vi "Car Wash New.vi"() -> ()   [LabVIEW 2021]
uses:
  Controls/Car Wash Indicators.ctl
  Controls/Wash Options.ctl
  Controls/Time.ctl
panel:
  in  "stop":bool
  in  "Start":bool
  out "Elapsed Time":dbl format="%0.2f"
  out "Wash Entry":bool
  in  "Wash Options":T1
  in  "Car Position Slider":i32(slide) max=3 scale=0.0..4.0
  out "Car Wash Indicators":T2
  # "Entry Console"
  # "Car Wash Display"
  # "Car Position Simulation"
  # "Pre-Soak\nH-P Wash\nL-P Wax\nSpot Free Rinse"
  # "Underbody Wash\nBug Remover"
  # "Tire Shine\nAir Dry"
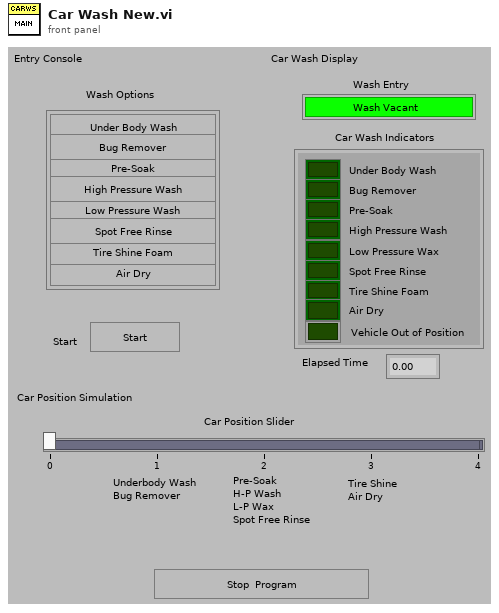
[diagram p1: front panel]
types:
  T1 = typedef "Wash Options.ctl" = cluster{"Underbody Wash":bool, "Bug Remover":bool, "Pre-Soak":bool, "High Pressure Wash":bool, "Low Pressure Wax":bool, "Spot Free Rinse":bool, "Tire Shine Foam":bool, "Air Dry":bool}
  T2 = typedef "Car Wash Indicators.ctl" = cluster{"Under Body Wash":bool, "Bug Remover":bool, "Pre-Soak":bool, "High Pressure Wash":bool, "Low Pressure Wax":bool, "Spot Free Rinse":bool, "Tire Shine Foam":bool, "Air Dry":bool, "Vehicle Out of Position":bool}
  T3 = enum32{"Invalid", "Standard", "Closed", "Hidden", "Minimized", "Maximized"}
  T4 = enum32{"invalid app kind", "Development System", "Run Time System", "Student Edition", "Embedded LabVIEW", "Evaluation", "Custom"}
  T5 = typedef "Time.ctl" = enum16{"Start", "Elapsed", "Pause", "int"}
  T6 = cluster{"Core":cluster{"Current VI Reference":refnum<vi>, "Close Panel on Exit?":bool}, "Your Boolean data":bool, "Your string data":string, "Wash Options":refnum<vi>, "Elapsed Time":refnum<vi>, "Car Position Slider":refnum<vi>, "Car Wash Indicators":refnum<vi>, "Wash Entry":refnum<vi>, "Time":dbl, "Car Wash Indicators":T2}
  T7 = cluster{"Current VI Reference":refnum<vi>, "Close Panel on Exit?":bool}
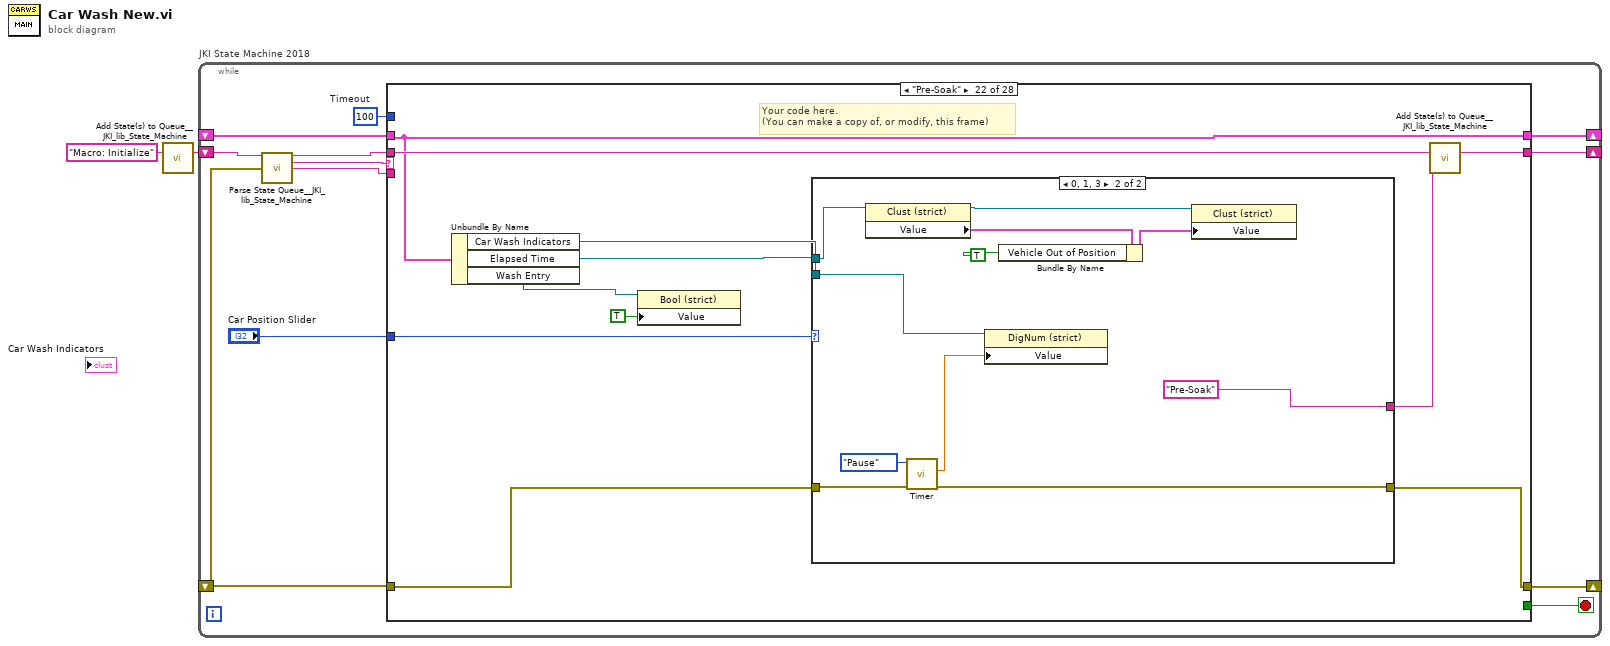
[diagram p0: block diagram]
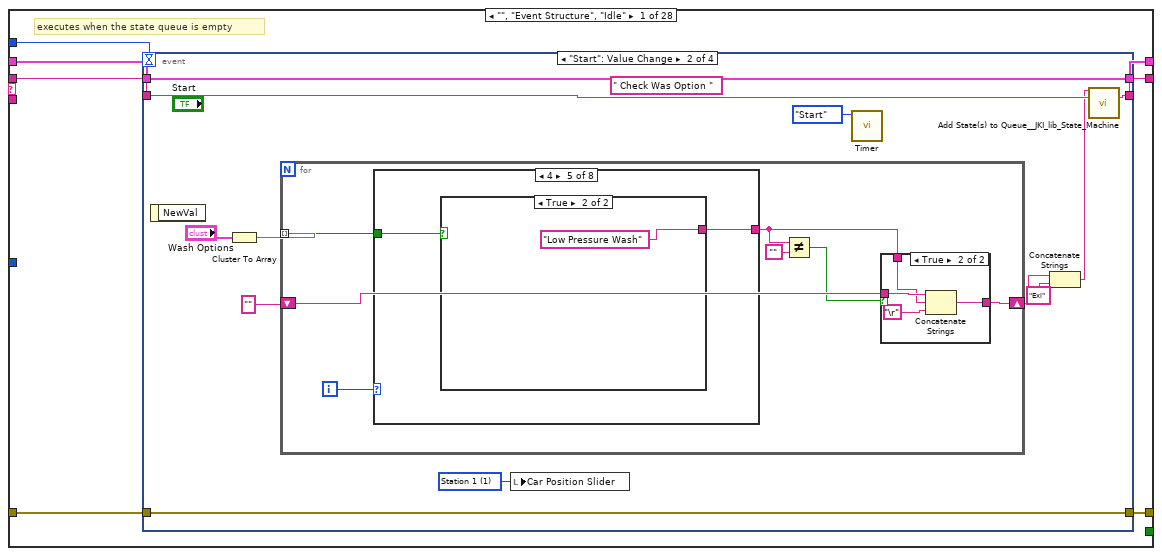
[diagram p2: hidden frame]
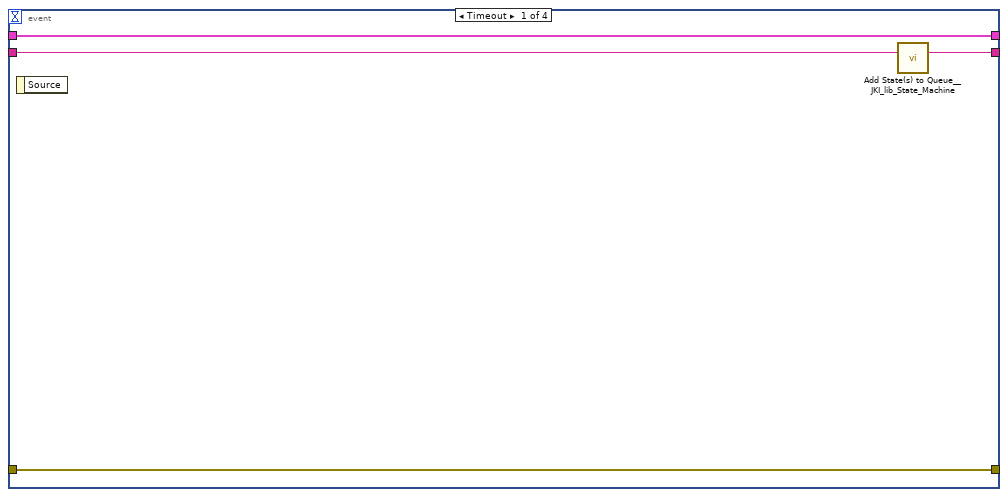
[diagram p3: hidden frame]
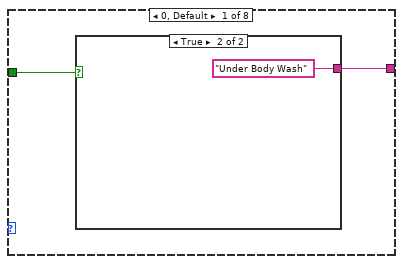
[diagram p5: hidden frame]
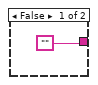
[diagram p6: hidden frame]
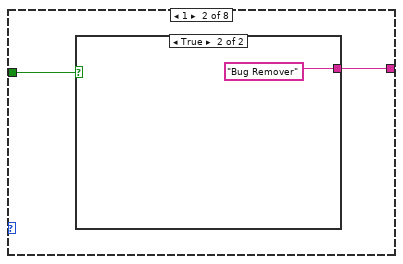
[diagram p7: hidden frame]
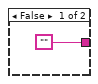
[diagram p8: hidden frame]
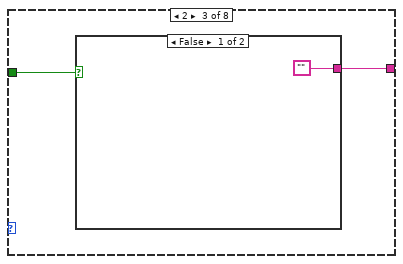
[diagram p9: hidden frame]
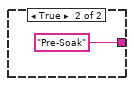
[diagram p10: hidden frame]
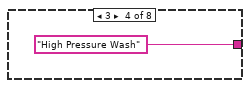
[diagram p11: hidden frame]
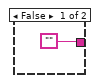
[diagram p12: hidden frame]
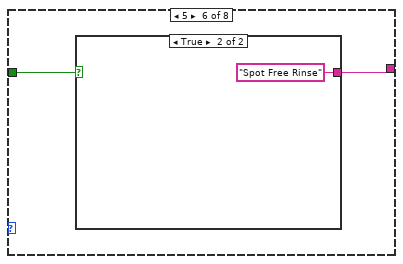
[diagram p13: hidden frame]
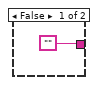
[diagram p14: hidden frame]
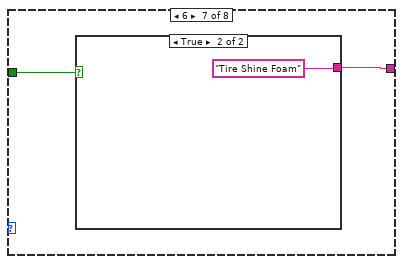
[diagram p15: hidden frame]
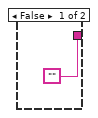
[diagram p16: hidden frame]
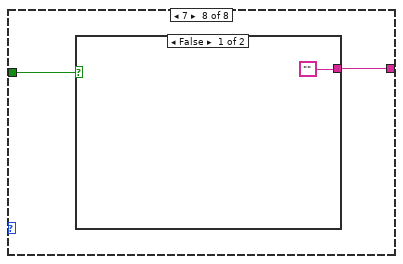
[diagram p17: hidden frame]
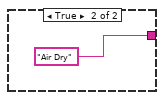
[diagram p18: hidden frame]
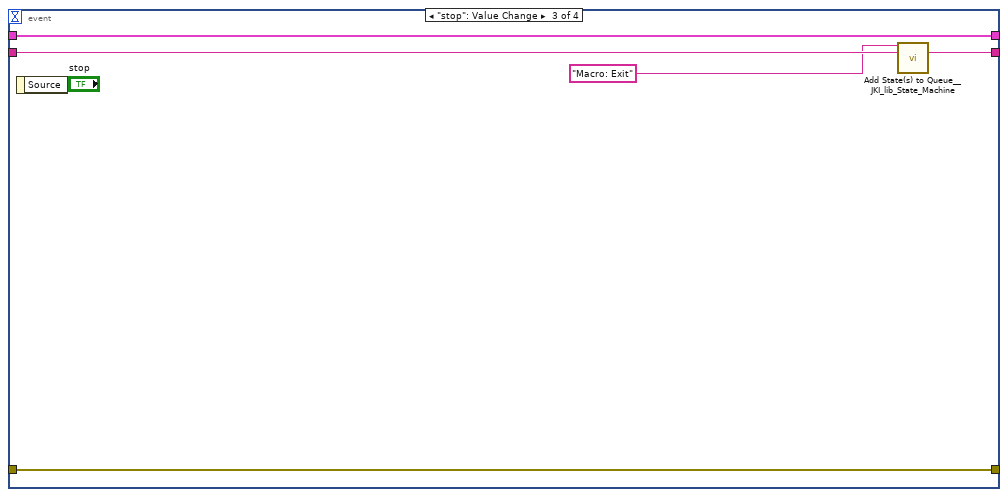
[diagram p19: hidden frame]
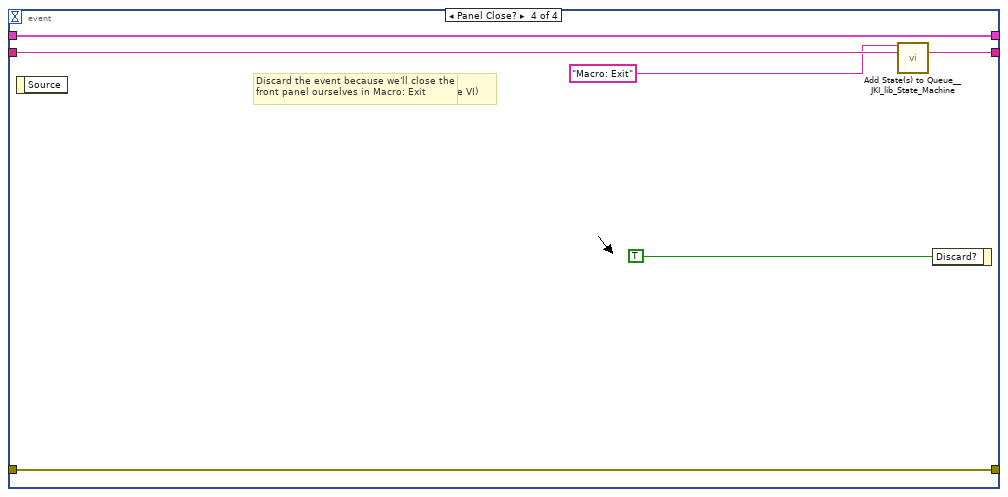
[diagram p20: hidden frame]
diagram:
  n1 = call <vilib>:"Add State(s) to Queue__JKI_lib_State_Machine.vi"("State(s) in (\"\")"="Macro: Initialize") -> ("States Out"=w2:string)  [unwired: 14 in]
  n2 = while "JKI State Machine 2018" {
    shift-right: [w7] -> _
    shift-left: _ -> [w3]
    shift-right: [w10] -> _
    shift-left: _ -> [w5]
    shift-right: [w9] -> _
    shift-left: w2 -> [w11]
    stop <- w8 stop-if-true
    w6 = 100  # Timeout
    n3 = call <vilib>:"Parse State Queue__JKI_lib_State_Machine.vi"("State Queue"=w11, "Error In (no error)"=w5) -> ("Remaining States"=w13:string, "Current State"=w14:string, "Arguments"=w12:string)  [unwired: 11 in]
    n4 = case shown="\"Pre-Soak\"" w14 {
      selector: w14 -> [_ _ w94 _ _ _ _ _ _ _ _ _ _ _ _ _ _ _ _ _ _ _ _ _ _ _ _ _]
      tunnel: w13 -> [w21 w93 w98 w117 w123 w128 w132 w148 w154 w158 w169 w175 w186 w255 w260 w270 w274 w278 w282 w293 w338 w383 w428 w473 w518 w563 w608 w652]
      tunnel: w12 -> [_ _ _ _ _ _ _ _ _ _ _ w170 w180 _ _ _ _ _ _ _ _ _ _ _ _ _ _ _]
      tunnel: w3 -> [w19 w90 w96 w110 w120 w126 w129 _ w149 w155 w160 w173 w182 w252 w257 w267 w271 w275 w279 w285 w330 w375 w420 w465 w510 w555 w600 w650]
      tunnel: [w18 w91 w100 w114 errorcluster {"status"=FALSE, "code"=0, "source"=""} ("error out") w125 w130 w145 w150 w156 w167 w171 w183 w253 w258 w268 w272 w276 w280 w288 w332 w380 w423 w469 w513 w558 w604 w647] -> w10
      tunnel: w5 -> [w17 w91 w99 w114 w119 w125 w130 w145 w151 w156 w167 w172 w184 w253 w258 w268 w272 w276 w280 w289 w333 w381 w425 w470 w514 w559 w605 w648]
      tunnel: [w20 w92 w97 w116 w122 w127 w131 w147 w153 w157 w168 w174 w185 w254 w259 w269 w273 w277 w281 w292 w337 w382 w427 w472 w517 w562 w607 w651] -> w9
      tunnel: [_ _ _ _ _ TRUE _ _ _ _ _ _ _ _ _ _ _ _ _ _ _ _ _ _ _ _ _ _] -> w8
      tunnel: [w16 w90 w96 w115 w120 w126 w129 w146 w149 w155 w160 w173 w182 w252 w257 w267 w271 w275 w279 w285 w330 w375 w420 w465 w510 w555 w600 w650] -> w7
      tunnel: w6 -> [w15 _ _ _ _ _ _ _ _ _ _ _ _ _ _ _ _ _ _ _ _ _ _ _ _ _ _ _]
      tunnel: "Car Position Slider" -> [_ _ _ _ _ _ _ _ _ _ _ _ _ _ _ _ _ _ _ w291 w334 w377 w422 w468 w515 w560 w603 w649]
      frame "", "Event Structure", "Idle" {
        # "executes when the state queue is empty"
        n5 = event shown="[1] \"Start\": Value Change" {
          selector: _ -> [_ _ _ _]
          dyn-events: _ -> [_ _ _ _]
          timeout: w15 -> [_ _ _ _]
          tunnel: w21 -> [w25 w37 w83 w89]
          tunnel: [w24 w36 w82 w88] -> w20
          tunnel: w19 -> [w22 w34 w80 w86]
          tunnel: [w23 w35 w81 w87] -> w18
          tunnel: w17 -> [w23 w35 w81 w87]
          tunnel: [w22 w34 w80 w86] -> w16
          event Timeout {
            n6 = event-data() -> ()  [unwired: 1 in, 1 out]
            n7 = call <vilib>:"Add State(s) to Queue__JKI_lib_State_Machine.vi"("State(s) in (\"\")"=w25) -> ("States Out"=w24:string)  [unwired: 14 in]
          }
          event "Start": Value Change {
            w26 = 1 items=["Entry", "Station 1", "Station 2", "Station 3", "Exit"] ("Car Position Slider")
            (unwired) " Check Was Option " ("State(s) at Back (\"\")")
            n8 = event-data() -> ()  [unwired: 1 in, 1 out]
            n9 = Cluster To Array(cluster="Wash Options") -> (array=w32:bool[])
            n10 = for {
              tunnel: w32 -> [w43] mode=indexing
              shift-right: [w42] -> w28
              shift-left: "" -> [w41]
              i -> [w44]
              n11 = case shown="4" w44 {
                tunnel: w43 -> [w51 w55 w59 _ w64 w68 w72 w76]
                tunnel: [w50 w54 w58 "High Pressure Wash" ("State(s) at Back (\"\")") w63 w67 w71 w75] -> w39
                frame 0, Default {
                  n12 = case shown="True" w51 {
                    tunnel: ["" "Under Body Wash" ("State(s) at Back (\"\")")] -> w50
                    frame False {
                    }
                    frame True {
                    }
                  }
                }
                frame 1 {
                  n13 = case shown="True" w55 {
                    tunnel: ["" "Bug Remover" ("State(s) at Back (\"\")")] -> w54
                    frame False {
                    }
                    frame True {
                    }
                  }
                }
                frame 2 {
                  n14 = case shown="False" w59 {
                    tunnel: ["" "Pre-Soak" ("State(s) at Back (\"\")")] -> w58
                    frame False {
                    }
                    frame True {
                    }
                  }
                }
                frame 3 {
                }
                frame 4 {
                  n15 = case shown="True" w64 {
                    tunnel: ["" "Low Pressure Wash" ("State(s) at Back (\"\")")] -> w63
                    frame False {
                    }
                    frame True {
                    }
                  }
                }
                frame 5 {
                  n16 = case shown="True" w68 {
                    tunnel: ["" "Spot Free Rinse"] -> w67
                    frame False {
                    }
                    frame True {
                    }
                  }
                }
                frame 6 {
                  n17 = case shown="True" w72 {
                    tunnel: ["" "Tire Shine Foam"] -> w71
                    frame False {
                    }
                    frame True {
                    }
                  }
                }
                frame 7 {
                  n18 = case shown="False" w76 {
                    tunnel: ["" "Air Dry"] -> w75
                    frame False {
                    }
                    frame True {
                    }
                  }
                }
              }
              n19 = Not Equal?(x=w39, y="") -> (x != y?=w38:bool)
              n20 = case shown="True" w38 {
                tunnel: [w45 w48] -> w42
                tunnel: w41 -> [w45 w47]
                tunnel: w39 -> [_ w46]
                frame False {
                }
                frame True {
                  n21 = Concatenate Strings(w47, w46, "\r") -> (w48:string)
                }
              }
            }
            n22 = local write "Car Position Slider"(w26) -> ()
            n23 = call "Timer.vi"("State"=enum16{"Start", "Elapsed", "Pause"}."Start") -> ()  [unwired: 8 in, 3 out]
            n24 = Concatenate Strings(w28, "Exi") -> (w27:string)
            n25 = call <vilib>:"Add State(s) to Queue__JKI_lib_State_Machine.vi"("State(s) in Front (\"\")"=w27, "State(s) in (\"\")"=w37) -> ("States Out"=w36:string)  [unwired: 13 in]
          }
          event "stop": Value Change {
            n26 = event-data() -> ()  [unwired: 1 in, 1 out]
            n27 = call <vilib>:"Add State(s) to Queue__JKI_lib_State_Machine.vi"("State(s) in Front (\"\")"="Macro: Exit", "State(s) in (\"\")"=w83) -> ("States Out"=w82:string)  [unwired: 13 in]
          }
          event Panel Close? {
            # "Discard the event because we'll close the front panel ourselves in Macro: Exit"
            # "Close Panel button (pressed) Event\n(this executes Macro: Exit to terminate the VI)"
            n28 = event-data() -> ()  [unwired: 1 in, 1 out]
            n29 = call <vilib>:"Add State(s) to Queue__JKI_lib_State_Machine.vi"("State(s) in Front (\"\")"="Macro: Exit", "State(s) in (\"\")"=w89) -> ("States Out"=w88:string)  [unwired: 13 in]
            n30 = event-data("Discard?"=TRUE) -> ()  [unwired: 1 in, 1 out]
          }
        }
      }
      frame "---------- Core ----------" {
        # "Do not put any code in this frame.\n(it is a separator no-op)"
        n31 = call <vilib>:"Add State(s) to Queue__JKI_lib_State_Machine.vi"("State(s) in (\"\")"=w93) -> ("States Out"=w92:string)  [unwired: 14 in]
      }
      frame Default {
        w103 = 42 items=["No error", "Argument error", "Memory is full", "Out of zone", "End of file", "File already open", "Generic file I/O error", "File not found", "File permission error", "Disk is full", "Duplicate path", "Too many files open", "System feature not enabled", "Resource file not found", "Cannot add resource", "Resource not found", "Image not found", "Image memory error", "Pen does not exist", "Config type invalid", "Config token not found", "Config parse error", "Config memory error", "Bad external code format", "Bad external code offset", "External code not present", "Null window", "Destroy window error", "Null menu", "Print aborted", "Bad print record", "Print driver error", "Windows error during printing", "Memory error during printing", "Print dialog error", "Generic print error", "Invalid device refnum", "Device not found", "Device parameter error", "Device unit error", "Cannot open device", "Device call aborted", "Generic error", "Cancelled by user", "Object ID too low", "Object ID too high", "Object not in heap", "Unknown heap", "Unknown object (invalid DefProc)", "Unknown object (DefProc not in table)", "Message out of range", "Invalid (null) method", "Unknown message", "Manager call not supported", "Bad address", "Network operation in progress", "Network operation timed out", "Connection is busy", "Network attribute not supported", "Network error", "Address in use", "System out of memory", "Connection aborted", "Connection refused", "Not connected", "Already connected", "Connection closed", "Initialization error (interapplication manager)", "Bad occurrence", "Wait on unbound occurrence handler", "Occurrence queue overflow", "Datalog type conflict", "Unused", "Unrecognized type (interapplication manager)", "Memory corrupt", "Failed to make temporary DLL", "Old CIN version", "Drag socket not found", "Failed to load drop-object", "Failed to register OLE object", "Failed to release OLE object", "Format specifier type mismatch", "Unknown format specifier", "Too few format specifiers", "Too many format specifiers", "Scan failed", "Newer CIN version", "Error converting to variant", "Runtime menu error", "Password tampered", "Variant attribute not found", "Incompatible variant data type", "Event data is not available", "Event Store is not present", "Occurrence is not found", "Event Queue is not created", "Event info is not available", "Refnum passed is NULL", "Error retrieving Class GUID", "Error retrieving CoClass GUID", "Error retrieving TypeLib GUID.", "Bad built application magic bytes.", "Specific driver is different from the specific driver associated with the Logical Name.", "There is no session opened to the class driver.", "Max Error", "MAX - Error with config objects", "MAX - Error loading configuration", "MAX - Group not supported"]
        # "Current State"
        # "Do not delete, rename, or modify this frame.\n(this is used to capture unhandled states and typos)"
        n32 = Format Into String(format string="Software Exception: Unhandled State \"%s\"." ("message"), error in=w99, w94) -> (resulting string=w102:string, error out=w101:errorcluster)  [unwired: 1 in]
        n33 = call <vilib>:"Error Cluster From Error Code.vi"("show call chain? (False)"=TRUE, "error in (no error)"=w101, "error message (\"\")"=w102, "error code (0)"=w103) -> ("error out"=w100:errorcluster)  [unwired: 5 in]
        n34 = call <vilib>:"Add State(s) to Queue__JKI_lib_State_Machine.vi"("State(s) in (\"\")"=w98) -> ("States Out"=w97:string)  [unwired: 14 in]
      }
      frame "Initialize Core Data" {
        # "Do not delete, rename, or modify this frame.\n(this is used to determine panel behavior on exit)"
        # "originally closed?"
        # "exe?"
        n35 = property class="VI"() -> ("FP.State"=w107:T3)  [unwired: 2 in, 2 out]
        n36 = property class="App"() -> ("App.Kind"=w113:T4)  [unwired: 2 in, 2 out]
        n37 = control-ref of="Current VI Reference"() -> (w108:refnum<vi>)
        n38 = Equal?(x=w107, y=T3."Closed" ("Front Panel Window:State")) -> (x = y?=w105:bool)
        n39 = Equal?(x=w113, y=T4."Run Time System" ("Application:Kind")) -> (x = y?=w111:bool)
        n40 = Or(x=w105, y=w111) -> (x .or. y?=w109:bool)
        n41 = Bundle By Name(cluster=w110, "Core.Current VI Reference"=w108, "Core.Close Panel on Exit?"=w109) -> (w115:T6)
        n42 = call <vilib>:"Add State(s) to Queue__JKI_lib_State_Machine.vi"("State(s) in (\"\")"=w117) -> ("States Out"=w116:string)  [unwired: 14 in]
      }
      frame "Error Handler" {
        # "Unhandled Error -- Display it"
        # "Handle any errors here.\nYou can also output any states to clean-up after errors occur"
        # "Clear error"
        n43 = call <vilib>:"General Error Handler.vi"("error in (no error)"=w119) -> ()  [unwired: 10 in, 5 out]
        n44 = call <vilib>:"Add State(s) to Queue__JKI_lib_State_Machine.vi"("State(s) in Front (\"\")"="/* Post Error States", "State(s) in (\"\")"=w123) -> ("States Out"=w122:string)  [unwired: 13 in]
      }
      frame "Exit" {
        # "Do not put any code in this frame.\n(No errors that occur here will be handled.)"
        n45 = call <vilib>:"Add State(s) to Queue__JKI_lib_State_Machine.vi"("State(s) in (\"\")"=w128) -> ("States Out"=w127:string)  [unwired: 14 in]
      }
      frame "---------- Data ----------" {
        # "Do not put any code in this frame.\n(It is a separator no-op. You can make a copy of this frame to create a new Data frame)"
        n46 = call <vilib>:"Add State(s) to Queue__JKI_lib_State_Machine.vi"("State(s) in (\"\")"=w132) -> ("States Out"=w131:string)  [unwired: 14 in]
      }
      frame "Data: Initialize" {
        w136 = 5.0  # Time
        w142 = T7 {"Current VI Reference"=refnum, "Close Panel on Exit?"=FALSE}  # Core
        w144 = TRUE  # Your Boolean data
        w143 = ""  # Your string data
        # "Initialize the shift-register data, here.\n(data names are defined by what you wire into the bundle function)"
        n47 = control-ref of="Elapsed Time"() -> (w141:refnum<vi>)
        n48 = control-ref of="Wash Options"() -> (w140:refnum<vi>)
        n49 = control-ref of="Car Position Slider"() -> (w139:refnum<vi>)
        n50 = control-ref of="Car Wash Indicators"() -> (w138:refnum<vi>)
        n51 = control-ref of="Wash Entry"() -> (w134:refnum<vi>)
        n52 = call "Timer.vi"("Timer (Sec)"=w136, "State"=Time."int") -> ()  [unwired: 7 in, 3 out]
        n53 = Bundle("Core"=w142, "Your Boolean data"=w144, "Your string data"=w143, "Wash Options"=w140, "Elapsed Time"=w141, "Car Position Slider"=w139, "Car Wash Indicators"=w138, "Wash Entry"=w134, "Time"=w136, "Car Wash Indicators"=T2 {"Under Body Wash"=FALSE, "Bug Remover"=FALSE, "Pre-Soak"=FALSE, "High Pressure Wash"=FALSE, "Low Pressure Wax"=FALSE, "Spot Free Rinse"=FALSE, "Tire Shine Foam"=FALSE, "Air Dry"=FALSE, "Vehicle Out of Position"=FALSE}) -> (w146:T6)  [unwired: 1 in]
        n54 = call <vilib>:"Add State(s) to Queue__JKI_lib_State_Machine.vi"("State(s) in (\"\")"=w148) -> ("States Out"=w147:string)  [unwired: 14 in]
        "Wash Entry" <- FALSE ("Wash Entry")
      }
      frame "Data: Cleanup" {
        # "Cleanup any data and references, here.\n(this is called automatically, by the Macro: Exit)"
        n55 = Unbundle By Name(w149) -> ("Core.Current VI Reference"=w152:refnum<vi>)
        n56 = Close Reference(reference=w152, error in (no error)=w151) -> (error out=w150:errorcluster)
        n57 = call <vilib>:"Add State(s) to Queue__JKI_lib_State_Machine.vi"("State(s) in (\"\")"=w154) -> ("States Out"=w153:string)  [unwired: 14 in]
      }
      frame "---------- UI ----------" {
        # "Do not put any code in this frame.\n(It is a separator no-op. You can make a copy of this frame to create a new UI frame)"
        n58 = call <vilib>:"Add State(s) to Queue__JKI_lib_State_Machine.vi"("State(s) in (\"\")"=w158) -> ("States Out"=w157:string)  [unwired: 14 in]
      }
      frame "UI: Initialize" {
        w159 = FALSE ("Car Wash Indicators.Under Body Wash")
        n59 = Unbundle By Name(w160) -> ("Car Wash Indicators"=w163:refnum<vi>, "Wash Entry"=w162:refnum<vi>)
        n60 = property class="Bool (strict)"(reference=w162, "Value"=FALSE) -> ()  [unwired: 1 in, 2 out]
        n61 = property class="Clust (strict)"(reference=w163) -> (reference out=w166:refnum<vi>, "Value"=w165:T2)  [unwired: 1 in, 1 out]
        n62 = Bundle By Name(cluster=w165, "Under Body Wash"=w159, "Bug Remover"=w159, "Pre-Soak"=w159, "High Pressure Wash"=w159, "Low Pressure Wax"=w159, "Spot Free Rinse"=w159, "Tire Shine Foam"=w159, "Air Dry"=w159, "Vehicle Out of Position"=w159) -> (w164:T2)
        n63 = property class="Clust (strict)"(reference=w166, "Value"=w164) -> ()  [unwired: 1 in, 2 out]
        n64 = call <vilib>:"Add State(s) to Queue__JKI_lib_State_Machine.vi"("State(s) in (\"\")"=w169) -> ("States Out"=w168:string)  [unwired: 14 in]
      }
      frame "UI: Cursor Set" {
        # "Argument"
        # "Set and Unset Cursor Busy.\n(Usage: \"UI: Cursor Set >> Busy|Idle\")"
        n65 = case shown="\"Idle\", Default" w170 {
          tunnel: w172 -> [w177 w179]
          tunnel: [w176 w178] -> w171
          frame "Idle", Default {
            n66 = call <vilib>:"Unset Busy.vi"("error in (no error)"=w177) -> ("error out"=w176:errorcluster)  [unwired: 10 in]
          }
          frame "Busy" {
            n67 = call <vilib>:"Set Busy.vi"("error in (no error)"=w179) -> ("error out"=w178:errorcluster)  [unwired: 9 in, 1 out]
          }
        }
        n68 = call <vilib>:"Add State(s) to Queue__JKI_lib_State_Machine.vi"("State(s) in (\"\")"=w175) -> ("States Out"=w174:string)  [unwired: 14 in]
      }
      frame "UI: Front Panel State" {
        # "Argument"
        # "Set Front Panel Open or Closed\n(Usage: \"UI: Front Panel State >> Open|Close\")"
        n69 = Unbundle By Name(w182) -> ("Core.Current VI Reference"=w181:refnum<vi>)
        n70 = case shown="\"Minimize\", \"Minimized\"" w180 {
          tunnel: w184 -> [w192 w207 w218 w231 w244]
          tunnel: [w194 w208 w220 w233 w246] -> w183
          tunnel: w181 -> [w193 w205 w219 w232 w245]
          frame "Open", "Standard", Default {
            w187 = T3."Standard" ("State")
            n71 = property class="VI"(reference=w193, error in=w192) -> (reference out=w190:refnum<vi>, error out=w191:errorcluster, "FP.State"=w189:T3)
            n72 = Not Equal?(x=w189, y=w187) -> (x != y?=w188:bool)
            n73 = case shown="True" w188 {
              tunnel: [w198 w200] -> w194
              tunnel: w191 -> [w197 w200]
              tunnel: w190 -> [w196 _]
              tunnel: w187 -> [w195 _]
              frame True {
                n74 = invoke class="VI" method="FP.Open"(reference=w196, error in=w197, "Activate"=TRUE, "State"=w195) -> (error out=w198:errorcluster)  [unwired: 1 in, 4 out]
              }
              frame False {
              }
            }
          }
          frame "Close", "Closed" {
            n75 = property class="VI"(reference=w205, error in=w207) -> (reference out=w204:refnum<vi>, error out=w206:errorcluster, "FP.State"=w202:T3)
            n76 = Not Equal?(x=w202, y=T3."Closed" ("Front Panel Window:State")) -> (x != y?=w201:bool)
            n77 = case shown="True" w201 {
              tunnel: [w209 w212] -> w208
              tunnel: w206 -> [w209 w211]
              tunnel: w204 -> [_ w210]
              frame False {
              }
              frame True {
                n78 = invoke class="VI" method="FP.Close"(reference=w210, error in=w211) -> (error out=w212:errorcluster)  [unwired: 1 in, 2 out]
              }
            }
          }
          frame "Hidden", "Hide" {
            w213 = T3."Hidden" ("State")
            n79 = property class="VI"(reference=w219, error in=w218) -> (reference out=w216:refnum<vi>, error out=w217:errorcluster, "FP.State"=w215:T3)
            n80 = Not Equal?(x=w215, y=w213) -> (x != y?=w214:bool)
            n81 = case shown="True" w214 {
              tunnel: [w224 w225] -> w220
              tunnel: w217 -> [w223 w225]
              tunnel: w216 -> [w222 _]
              tunnel: w213 -> [w221 _]
              frame True {
                n82 = invoke class="VI" method="FP.Open"(reference=w222, error in=w223, "State"=w221) -> (error out=w224:errorcluster)  [unwired: 2 in, 4 out]
              }
              frame False {
              }
            }
          }
          frame "Minimize", "Minimized" {
            w226 = T3."Minimized" ("State")
            n83 = property class="VI"(reference=w232, error in=w231) -> (reference out=w229:refnum<vi>, error out=w230:errorcluster, "FP.State"=w228:T3)
            n84 = Not Equal?(x=w228, y=w226) -> (x != y?=w227:bool)
            n85 = case shown="True" w227 {
              tunnel: [w237 w238] -> w233
              tunnel: w230 -> [w236 w238]
              tunnel: w229 -> [w235 _]
              tunnel: w226 -> [w234 _]
              frame True {
                n86 = invoke class="VI" method="FP.Open"(reference=w235, error in=w236, "State"=w234) -> (error out=w237:errorcluster)  [unwired: 2 in, 4 out]
              }
              frame False {
              }
            }
          }
          frame "Maximize", "Maximized" {
            w239 = T3."Maximized" ("State")
            n87 = property class="VI"(reference=w245, error in=w244) -> (reference out=w242:refnum<vi>, error out=w243:errorcluster, "FP.State"=w241:T3)
            n88 = Not Equal?(x=w241, y=w239) -> (x != y?=w240:bool)
            n89 = case shown="True" w240 {
              tunnel: [w250 w251] -> w246
              tunnel: w243 -> [w249 w251]
              tunnel: w242 -> [w248 _]
              tunnel: w239 -> [w247 _]
              frame True {
                n90 = invoke class="VI" method="FP.Open"(reference=w248, error in=w249, "State"=w247) -> (error out=w250:errorcluster)  [unwired: 2 in, 4 out]
              }
              frame False {
              }
            }
          }
        }
        n91 = call <vilib>:"Add State(s) to Queue__JKI_lib_State_Machine.vi"("State(s) in (\"\")"=w186) -> ("States Out"=w185:string)  [unwired: 14 in]
      }
      frame "---------- Macro ----------" {
        # "Do not put any code in this frame.\n(It is a separator no-op. You can make a copy of this frame to create a new Macro frame)"
        n92 = call <vilib>:"Add State(s) to Queue__JKI_lib_State_Machine.vi"("State(s) in (\"\")"=w255) -> ("States Out"=w254:string)  [unwired: 14 in]
      }
      frame "Macro: Initialize" {
        w256 = "Data: Initialize\nInitialize Core Data\nUI: Initialize\nUI: Front Panel State >> Open"  # Data: Initialize Initialize Core Data UI: Initialize UI: Front Panel State >> Open
        # "Initialization Macro\n(This is called once, when the VI starts)"
        n93 = call <vilib>:"Add State(s) to Queue__JKI_lib_State_Machine.vi"("State(s) in Front (\"\")"=w256, "State(s) in (\"\")"=w260) -> ("States Out"=w259:string)  [unwired: 13 in]
      }
      frame "Macro: Exit" {
        # "Exit Macro\n(This is called once, when the VI exits)"
        n94 = Unbundle By Name(w267) -> ("Core.Close Panel on Exit?"=w266:bool)
        n95 = Select(t="UI: Front Panel State >> Close", s=w266, f="") -> (s? t:f=w263:string)
        n96 = call <vilib>:"Add State(s) to Queue__JKI_lib_State_Machine.vi"("State(s) in (\"\")"=w263, "State(s) at Back (\"\")"="Data: Cleanup\nExit") -> ("States Out"=w261:string)  [unwired: 13 in]
        n97 = call <vilib>:"Add State(s) to Queue__JKI_lib_State_Machine.vi"("State(s) in Front (\"\")"=w261, "State(s) in (\"\")"=w270) -> ("States Out"=w269:string)  [unwired: 13 in]
      }
      frame "---------- New Category ----------" {
        # "Template Separator\n(You can make a copy of, or modify, this frame)"
        n98 = call <vilib>:"Add State(s) to Queue__JKI_lib_State_Machine.vi"("State(s) in (\"\")"=w274) -> ("States Out"=w273:string)  [unwired: 14 in]
      }
      frame "New Category: 1" {
        # "Your code here.\n(You can make a copy of, or modify, this frame)"
        n99 = call <vilib>:"Add State(s) to Queue__JKI_lib_State_Machine.vi"("State(s) in (\"\")"=w278) -> ("States Out"=w277:string)  [unwired: 14 in]
      }
      frame "New Category: 2" {
        # "Your code here.\n(You can make a copy of, or modify, this frame)"
        n100 = call <vilib>:"Add State(s) to Queue__JKI_lib_State_Machine.vi"("State(s) in (\"\")"=w282) -> ("States Out"=w281:string)  [unwired: 14 in]
      }
      frame "Under Body Wash" {
        # "Your code here.\n(You can make a copy of, or modify, this frame)"
        n101 = Unbundle By Name(w285) -> ("Car Wash Indicators"=w286:refnum<vi>, "Elapsed Time"=w290:refnum<vi>, "Wash Entry"=w283:refnum<vi>)
        n102 = property class="Bool (strict)"(reference=w283, "Value"=TRUE) -> ()  [unwired: 1 in, 2 out]
        n103 = case shown="1, Default" w291 {
          tunnel: [w306 w322] -> w288
          tunnel: w290 -> [w301 w326]
          tunnel: [w303 "Under Body Wash"] -> w287
          tunnel: w289 -> [w302 w323]
          tunnel: w286 -> [w297 w320]
          frame 1, Default {
            n104 = property class="Clust (strict)"(reference=w297) -> (reference out=w294:refnum<vi>, "Value"=w296:T2)  [unwired: 1 in, 1 out]
            n105 = call "Timer.vi"("entrée d'erreur"=w302, "State"=Time."Elapsed") -> ("sortie d'erreur"=w307:errorcluster, "Elapsed"=w300:dbl, "Elapsed?"=w308:bool)  [unwired: 7 in]
            n106 = property class="DigNum (strict)"(reference=w301, "Value"=w300) -> (reference out=w299:refnum<vi>)  [unwired: 1 in, 1 out]
            n107 = Bundle By Name(cluster=w296, "Vehicle Out of Position"=FALSE, "Under Body Wash"=TRUE) -> (w295:T2)
            n108 = case shown="False" w308 {
              tunnel: w307 -> [w310 w316]
              tunnel: [w310 w315] -> w306
              tunnel: ["Under Body Wash" ""] -> w303
              tunnel: w299 -> [_ w312]
              frame False {
              }
              frame True {
                n109 = call "Timer.vi"("entrée d'erreur"=w316, "State"=Time."Start") -> ("sortie d'erreur"=w315:errorcluster, "Elapsed"=w313:dbl)  [unwired: 7 in, 1 out]
                n110 = property class="DigNum (strict)"(reference=w312, "Value"=w313) -> ()  [unwired: 1 in, 2 out]
              }
            }
            n111 = property on="Property Node" class="Clust (strict)"(reference=w294, "Value"=w295) -> ()  [unwired: 1 in, 2 out]
          }
          frame 0, 2, 3 {
            n112 = property class="Clust (strict)"(reference=w320) -> (reference out=w317:refnum<vi>, "Value"=w319:T2)  [unwired: 1 in, 1 out]
            n113 = call "Timer.vi"("entrée d'erreur"=w323, "State"=Time."Pause") -> ("sortie d'erreur"=w322:errorcluster, "Elapsed"=w325:dbl)  [unwired: 7 in, 1 out]
            n114 = property class="DigNum (strict)"(reference=w326, "Value"=w325) -> ()  [unwired: 1 in, 2 out]
            n115 = Bundle By Name(cluster=w319, "Vehicle Out of Position"=TRUE) -> (w318:T2)
            n116 = property class="Clust (strict)"(reference=w317, "Value"=w318) -> ()  [unwired: 1 in, 2 out]
          }
        }
        n117 = call <vilib>:"Add State(s) to Queue__JKI_lib_State_Machine.vi"("State(s) in Front (\"\")"=w287, "State(s) in (\"\")"=w293) -> ("States Out"=w292:string)  [unwired: 13 in]
      }
      frame "Bug Remover" {
        # "Your code here.\n(You can make a copy of, or modify, this frame)"
        n118 = Unbundle By Name(w330) -> ("Car Wash Indicators"=w331:refnum<vi>, "Elapsed Time"=w335:refnum<vi>, "Wash Entry"=w328:refnum<vi>)
        n119 = property class="Bool (strict)"(reference=w328, "Value"=TRUE) -> ()  [unwired: 1 in, 2 out]
        n120 = case shown="1, Default" w334 {
          tunnel: [w351 w368] -> w332
          tunnel: w335 -> [w346 w372]
          tunnel: [w348 "Bug Remover"] -> w336
          tunnel: w333 -> [w347 w369]
          tunnel: w331 -> [w342 w362]
          frame 1, Default {
            n121 = call "Timer.vi"("entrée d'erreur"=w347, "State"=Time."Elapsed") -> ("sortie d'erreur"=w352:errorcluster, "Elapsed"=w344:dbl, "Elapsed?"=w353:bool)  [unwired: 7 in]
            n122 = property class="Clust (strict)"(reference=w342) -> (reference out=w339:refnum<vi>, "Value"=w341:T2)  [unwired: 1 in, 1 out]
            n123 = property class="DigNum (strict)"(reference=w346, "Value"=w344) -> (reference out=w345:refnum<vi>)  [unwired: 1 in, 1 out]
            n124 = Bundle By Name(cluster=w341, "Vehicle Out of Position"=FALSE, "Bug Remover"=TRUE ("Under Body Wash")) -> (w340:T2)
            n125 = case shown="True" w353 {
              tunnel: w352 -> [w354 w361]
              tunnel: [w354 w360] -> w351
              tunnel: ["Bug Remover" ""] -> w348
              tunnel: w345 -> [_ w357]
              frame False {
              }
              frame True {
                n126 = call "Timer.vi"("entrée d'erreur"=w361, "State"=Time."Start") -> ("sortie d'erreur"=w360:errorcluster, "Elapsed"=w358:dbl)  [unwired: 7 in, 1 out]
                n127 = property class="DigNum (strict)"(reference=w357, "Value"=w358) -> ()  [unwired: 1 in, 2 out]
              }
            }
            n128 = property class="Clust (strict)"(reference=w339, "Value"=w340) -> ()  [unwired: 1 in, 2 out]
          }
          frame 0, 2, 3 {
            n129 = property class="Clust (strict)"(reference=w362) -> (reference out=w363:refnum<vi>, "Value"=w365:T2)  [unwired: 1 in, 1 out]
            n130 = call "Timer.vi"("entrée d'erreur"=w369, "State"=Time."Pause") -> ("sortie d'erreur"=w368:errorcluster, "Elapsed"=w371:dbl)  [unwired: 7 in, 1 out]
            n131 = Bundle By Name(cluster=w365, "Vehicle Out of Position"=TRUE) -> (w364:T2)
            n132 = property class="DigNum (strict)"(reference=w372, "Value"=w371) -> ()  [unwired: 1 in, 2 out]
            n133 = property class="Clust (strict)"(reference=w363, "Value"=w364) -> ()  [unwired: 1 in, 2 out]
          }
        }
        n134 = call <vilib>:"Add State(s) to Queue__JKI_lib_State_Machine.vi"("State(s) in Front (\"\")"=w336, "State(s) in (\"\")"=w338) -> ("States Out"=w337:string)  [unwired: 13 in]
      }
      frame "Pre-Soak" {
        # "Your code here.\n(You can make a copy of, or modify, this frame)"
        n135 = Unbundle By Name(w375) -> ("Car Wash Indicators"=w376:refnum<vi>, "Elapsed Time"=w378:refnum<vi>, "Wash Entry"=w373:refnum<vi>)
        n136 = property class="Bool (strict)"(reference=w373, "Value"=TRUE) -> ()  [unwired: 1 in, 2 out]
        n137 = case shown="0, 1, 3" w377 {
          tunnel: [w396 w413] -> w380
          tunnel: w378 -> [w390 w417]
          tunnel: [w393 "Pre-Soak"] -> w379
          tunnel: w381 -> [w392 w414]
          tunnel: w376 -> [w387 w407]
          frame 2, Default {
            n138 = property class="Clust (strict)"(reference=w387) -> (reference out=w384:refnum<vi>, "Value"=w386:T2)  [unwired: 1 in, 1 out]
            n139 = call "Timer.vi"("entrée d'erreur"=w392, "State"=Time."Elapsed") -> ("sortie d'erreur"=w397:errorcluster, "Elapsed"=w388:dbl, "Elapsed?"=w398:bool)  [unwired: 7 in]
            n140 = property class="DigNum (strict)"(reference=w390, "Value"=w388) -> (reference out=w389:refnum<vi>)  [unwired: 1 in, 1 out]
            n141 = Bundle By Name(cluster=w386, "Vehicle Out of Position"=FALSE, "Pre-Soak"=TRUE ("Under Body Wash")) -> (w385:T2)
            n142 = case shown="False" w398 {
              tunnel: w397 -> [w399 w406]
              tunnel: [w399 w405] -> w396
              tunnel: ["Pre-Soak" ""] -> w393
              tunnel: w389 -> [_ w402]
              frame False {
              }
              frame True {
                n143 = call "Timer.vi"("entrée d'erreur"=w406, "State"=Time."Start") -> ("sortie d'erreur"=w405:errorcluster, "Elapsed"=w403:dbl)  [unwired: 7 in, 1 out]
                n144 = property class="DigNum (strict)"(reference=w402, "Value"=w403) -> ()  [unwired: 1 in, 2 out]
              }
            }
            n145 = property class="Clust (strict)"(reference=w384, "Value"=w385) -> ()  [unwired: 1 in, 2 out]
          }
          frame 0, 1, 3 {
            n146 = property class="Clust (strict)"(reference=w407) -> (reference out=w408:refnum<vi>, "Value"=w410:T2)  [unwired: 1 in, 1 out]
            n147 = call "Timer.vi"("entrée d'erreur"=w414, "State"=Time."Pause") -> ("sortie d'erreur"=w413:errorcluster, "Elapsed"=w416:dbl)  [unwired: 7 in, 1 out]
            n148 = property class="DigNum (strict)"(reference=w417, "Value"=w416) -> ()  [unwired: 1 in, 2 out]
            n149 = Bundle By Name(cluster=w410, "Vehicle Out of Position"=TRUE) -> (w409:T2)
            n150 = property class="Clust (strict)"(reference=w408, "Value"=w409) -> ()  [unwired: 1 in, 2 out]
          }
        }
        n151 = call <vilib>:"Add State(s) to Queue__JKI_lib_State_Machine.vi"("State(s) in Front (\"\")"=w379, "State(s) in (\"\")"=w383) -> ("States Out"=w382:string)  [unwired: 13 in]
      }
      frame "High Pressure Wash" {
        # "Your code here.\n(You can make a copy of, or modify, this frame)"
        n152 = Unbundle By Name(w420) -> ("Car Wash Indicators"=w421:refnum<vi>, "Elapsed Time"=w426:refnum<vi>, "Wash Entry"=w418:refnum<vi>)
        n153 = property class="Bool (strict)"(reference=w418, "Value"=TRUE) -> ()  [unwired: 1 in, 2 out]
        n154 = case shown="2, Default" w422 {
          tunnel: [w441 w458] -> w423
          tunnel: w426 -> [w437 w462]
          tunnel: [w440 "High Pressure Wash"] -> w424
          tunnel: w425 -> [w439 w459]
          tunnel: w421 -> [w429 w452]
          frame 2, Default {
            n155 = property class="Clust (strict)"(reference=w429) -> (reference out=w430:refnum<vi>, "Value"=w432:T2)  [unwired: 1 in, 1 out]
            n156 = call "Timer.vi"("entrée d'erreur"=w439, "State"=Time."Elapsed") -> ("sortie d'erreur"=w442:errorcluster, "Elapsed"=w435:dbl, "Elapsed?"=w443:bool)  [unwired: 7 in]
            n157 = property class="DigNum (strict)"(reference=w437, "Value"=w435) -> (reference out=w436:refnum<vi>)  [unwired: 1 in, 1 out]
            n158 = Bundle By Name(cluster=w432, "Vehicle Out of Position"=FALSE, "High Pressure Wash"=TRUE ("Under Body Wash")) -> (w431:T2)
            n159 = case shown="True" w443 {
              tunnel: w442 -> [w444 w451]
              tunnel: [w444 w450] -> w441
              tunnel: ["High Pressure Wash" ""] -> w440
              tunnel: w436 -> [_ w447]
              frame False {
              }
              frame True {
                n160 = call "Timer.vi"("entrée d'erreur"=w451, "State"=Time."Start") -> ("sortie d'erreur"=w450:errorcluster, "Elapsed"=w448:dbl)  [unwired: 7 in, 1 out]
                n161 = property class="DigNum (strict)"(reference=w447, "Value"=w448) -> ()  [unwired: 1 in, 2 out]
              }
            }
            n162 = property class="Clust (strict)"(reference=w430, "Value"=w431) -> ()  [unwired: 1 in, 2 out]
          }
          frame 0, 1, 3 {
            n163 = property class="Clust (strict)"(reference=w452) -> (reference out=w453:refnum<vi>, "Value"=w455:T2)  [unwired: 1 in, 1 out]
            n164 = call "Timer.vi"("entrée d'erreur"=w459, "State"=Time."Pause") -> ("sortie d'erreur"=w458:errorcluster, "Elapsed"=w461:dbl)  [unwired: 7 in, 1 out]
            n165 = Bundle By Name(cluster=w455, "Vehicle Out of Position"=TRUE) -> (w454:T2)
            n166 = property class="DigNum (strict)"(reference=w462, "Value"=w461) -> ()  [unwired: 1 in, 2 out]
            n167 = property class="Clust (strict)"(reference=w453, "Value"=w454) -> ()  [unwired: 1 in, 2 out]
          }
        }
        n168 = call <vilib>:"Add State(s) to Queue__JKI_lib_State_Machine.vi"("State(s) in Front (\"\")"=w424, "State(s) in (\"\")"=w428) -> ("States Out"=w427:string)  [unwired: 13 in]
      }
      frame "Low Pressure Wash" {
        # "Your code here.\n(You can make a copy of, or modify, this frame)"
        n169 = Unbundle By Name(w465) -> ("Car Wash Indicators"=w466:refnum<vi>, "Elapsed Time"=w471:refnum<vi>, "Wash Entry"=w463:refnum<vi>)
        n170 = property class="Bool (strict)"(reference=w463, "Value"=TRUE) -> ()  [unwired: 1 in, 2 out]
        n171 = case shown="2, Default" w468 {
          tunnel: [w486 w503] -> w469
          tunnel: w471 -> [w482 w507]
          tunnel: [w485 "Low Pressure Wash"] -> w467
          tunnel: w470 -> [w484 w504]
          tunnel: w466 -> [w474 w497]
          frame 2, Default {
            n172 = call "Timer.vi"("entrée d'erreur"=w484, "State"=Time."Elapsed") -> ("sortie d'erreur"=w487:errorcluster, "Elapsed"=w483:dbl, "Elapsed?"=w488:bool)  [unwired: 7 in]
            n173 = property class="Clust (strict)"(reference=w474) -> (reference out=w475:refnum<vi>, "Value"=w477:T2)  [unwired: 1 in, 1 out]
            n174 = property class="DigNum (strict)"(reference=w482, "Value"=w483) -> (reference out=w481:refnum<vi>)  [unwired: 1 in, 1 out]
            n175 = Bundle By Name(cluster=w477, "Vehicle Out of Position"=FALSE, "Low Pressure Wax"=TRUE ("Under Body Wash")) -> (w476:T2)
            n176 = case shown="False" w488 {
              tunnel: w487 -> [w489 w496]
              tunnel: [w489 w495] -> w486
              tunnel: ["Low Pressure Wash" ""] -> w485
              tunnel: w481 -> [_ w491]
              frame False {
              }
              frame True {
                n177 = call "Timer.vi"("entrée d'erreur"=w496, "State"=Time."Start") -> ("sortie d'erreur"=w495:errorcluster, "Elapsed"=w493:dbl)  [unwired: 7 in, 1 out]
                n178 = property class="DigNum (strict)"(reference=w491, "Value"=w493) -> ()  [unwired: 1 in, 2 out]
              }
            }
            n179 = property class="Clust (strict)"(reference=w475, "Value"=w476) -> ()  [unwired: 1 in, 2 out]
          }
          frame 0, 1, 3 {
            n180 = property class="Clust (strict)"(reference=w497) -> (reference out=w498:refnum<vi>, "Value"=w500:T2)  [unwired: 1 in, 1 out]
            n181 = call "Timer.vi"("entrée d'erreur"=w504, "State"=Time."Pause") -> ("sortie d'erreur"=w503:errorcluster, "Elapsed"=w506:dbl)  [unwired: 7 in, 1 out]
            n182 = Bundle By Name(cluster=w500, "Vehicle Out of Position"=TRUE) -> (w499:T2)
            n183 = property class="DigNum (strict)"(reference=w507, "Value"=w506) -> ()  [unwired: 1 in, 2 out]
            n184 = property class="Clust (strict)"(reference=w498, "Value"=w499) -> ()  [unwired: 1 in, 2 out]
          }
        }
        n185 = call <vilib>:"Add State(s) to Queue__JKI_lib_State_Machine.vi"("State(s) in Front (\"\")"=w467, "State(s) in (\"\")"=w473) -> ("States Out"=w472:string)  [unwired: 13 in]
      }
      frame "Spot Free Rinse" {
        # "Your code here.\n(You can make a copy of, or modify, this frame)"
        n186 = Unbundle By Name(w510) -> ("Car Wash Indicators"=w511:refnum<vi>, "Elapsed Time"=w516:refnum<vi>, "Wash Entry"=w508:refnum<vi>)
        n187 = property class="Bool (strict)"(reference=w508, "Value"=TRUE) -> ()  [unwired: 1 in, 2 out]
        n188 = case shown="2, Default" w515 {
          tunnel: [w531 w548] -> w513
          tunnel: w516 -> [w526 w552]
          tunnel: [w530 "Spot Free Rinse"] -> w512
          tunnel: w514 -> [w529 w549]
          tunnel: w511 -> [w519 w542]
          frame 2, Default {
            n189 = property class="Clust (strict)"(reference=w519) -> (reference out=w520:refnum<vi>, "Value"=w522:T2)  [unwired: 1 in, 1 out]
            n190 = call "Timer.vi"("entrée d'erreur"=w529, "State"=Time."Elapsed") -> ("sortie d'erreur"=w532:errorcluster, "Elapsed"=w527:dbl, "Elapsed?"=w533:bool)  [unwired: 7 in]
            n191 = property class="DigNum (strict)"(reference=w526, "Value"=w527) -> (reference out=w525:refnum<vi>)  [unwired: 1 in, 1 out]
            n192 = Bundle By Name(cluster=w522, "Vehicle Out of Position"=FALSE, "Spot Free Rinse"=TRUE ("Under Body Wash")) -> (w521:T2)
            n193 = case shown="True" w533 {
              tunnel: w532 -> [w534 w541]
              tunnel: [w534 w540] -> w531
              tunnel: ["Spot Free Rinse" ""] -> w530
              tunnel: w525 -> [_ w536]
              frame False {
              }
              frame True {
                n194 = call "Timer.vi"("entrée d'erreur"=w541, "State"=Time."Start") -> ("sortie d'erreur"=w540:errorcluster, "Elapsed"=w538:dbl)  [unwired: 7 in, 1 out]
                n195 = property class="DigNum (strict)"(reference=w536, "Value"=w538) -> ()  [unwired: 1 in, 2 out]
              }
            }
            n196 = property class="Clust (strict)"(reference=w520, "Value"=w521) -> ()  [unwired: 1 in, 2 out]
          }
          frame 0, 1, 3 {
            n197 = property class="Clust (strict)"(reference=w542) -> (reference out=w543:refnum<vi>, "Value"=w545:T2)  [unwired: 1 in, 1 out]
            n198 = call "Timer.vi"("entrée d'erreur"=w549, "State"=Time."Start") -> ("sortie d'erreur"=w548:errorcluster, "Elapsed"=w551:dbl)  [unwired: 7 in, 1 out]
            n199 = Bundle By Name(cluster=w545, "Vehicle Out of Position"=TRUE) -> (w544:T2)
            n200 = property class="DigNum (strict)"(reference=w552, "Value"=w551) -> ()  [unwired: 1 in, 2 out]
            n201 = property class="Clust (strict)"(reference=w543, "Value"=w544) -> ()  [unwired: 1 in, 2 out]
          }
        }
        n202 = call <vilib>:"Add State(s) to Queue__JKI_lib_State_Machine.vi"("State(s) in Front (\"\")"=w512, "State(s) in (\"\")"=w518) -> ("States Out"=w517:string)  [unwired: 13 in]
      }
      frame "Tire Shine Foam" {
        # "Your code here.\n(You can make a copy of, or modify, this frame)"
        n203 = Unbundle By Name(w555) -> ("Car Wash Indicators"=w556:refnum<vi>, "Elapsed Time"=w561:refnum<vi>, "Wash Entry"=w553:refnum<vi>)
        n204 = property class="Bool (strict)"(reference=w553, "Value"=TRUE) -> ()  [unwired: 1 in, 2 out]
        n205 = case shown="3, Default" w560 {
          tunnel: [w576 w593] -> w558
          tunnel: w561 -> [w573 w597]
          tunnel: [w575 "Tire Shine Foam"] -> w557
          tunnel: w559 -> [w574 w594]
          tunnel: w556 -> [w564 w587]
          frame 3, Default {
            n206 = property class="Clust (strict)"(reference=w564) -> (reference out=w565:refnum<vi>, "Value"=w567:T2)  [unwired: 1 in, 1 out]
            n207 = call "Timer.vi"("entrée d'erreur"=w574, "State"=Time."Elapsed") -> ("sortie d'erreur"=w577:errorcluster, "Elapsed"=w572:dbl, "Elapsed?"=w578:bool)  [unwired: 7 in]
            n208 = Bundle By Name(cluster=w567, "Vehicle Out of Position"=FALSE, "Tire Shine Foam"=TRUE ("Under Body Wash")) -> (w566:T2)
            n209 = property class="DigNum (strict)"(reference=w573, "Value"=w572) -> (reference out=w571:refnum<vi>)  [unwired: 1 in, 1 out]
            n210 = case shown="False" w578 {
              tunnel: w577 -> [w579 w586]
              tunnel: [w579 w585] -> w576
              tunnel: ["Tire Shine Foam" ""] -> w575
              tunnel: w571 -> [_ w582]
              frame False {
              }
              frame True {
                n211 = call "Timer.vi"("entrée d'erreur"=w586, "State"=Time."Start") -> ("sortie d'erreur"=w585:errorcluster, "Elapsed"=w583:dbl)  [unwired: 7 in, 1 out]
                n212 = property class="DigNum (strict)"(reference=w582, "Value"=w583) -> ()  [unwired: 1 in, 2 out]
              }
            }
            n213 = property class="Clust (strict)"(reference=w565, "Value"=w566) -> ()  [unwired: 1 in, 2 out]
          }
          frame 0..2 {
            n214 = property class="Clust (strict)"(reference=w587) -> (reference out=w588:refnum<vi>, "Value"=w590:T2)  [unwired: 1 in, 1 out]
            n215 = Bundle By Name(cluster=w590, "Vehicle Out of Position"=TRUE) -> (w589:T2)
            n216 = call "Timer.vi"("entrée d'erreur"=w594, "State"=Time."Pause") -> ("sortie d'erreur"=w593:errorcluster, "Elapsed"=w596:dbl)  [unwired: 7 in, 1 out]
            n217 = property class="DigNum (strict)"(reference=w597, "Value"=w596) -> ()  [unwired: 1 in, 2 out]
            n218 = property class="Clust (strict)"(reference=w588, "Value"=w589) -> ()  [unwired: 1 in, 2 out]
          }
        }
        n219 = call <vilib>:"Add State(s) to Queue__JKI_lib_State_Machine.vi"("State(s) in Front (\"\")"=w557, "State(s) in (\"\")"=w563) -> ("States Out"=w562:string)  [unwired: 13 in]
      }
      frame "Air Dry" {
        # "Your code here.\n(You can make a copy of, or modify, this frame)"
        n220 = Unbundle By Name(w600) -> ("Car Wash Indicators"=w601:refnum<vi>, "Elapsed Time"=w606:refnum<vi>, "Wash Entry"=w598:refnum<vi>)
        n221 = property class="Bool (strict)"(reference=w598, "Value"=TRUE) -> ()  [unwired: 1 in, 2 out]
        n222 = case shown="3, Default" w603 {
          tunnel: [w621 w638] -> w604
          tunnel: w606 -> [w617 w642]
          tunnel: [w620 "Air Dry"] -> w602
          tunnel: w605 -> [w619 w639]
          tunnel: w601 -> [w609 w632]
          frame 3, Default {
            n223 = call "Timer.vi"("entrée d'erreur"=w619, "State"=Time."Elapsed") -> ("sortie d'erreur"=w622:errorcluster, "Elapsed"=w616:dbl, "Elapsed?"=w623:bool)  [unwired: 7 in]
            n224 = property class="Clust (strict)"(reference=w609) -> (reference out=w610:refnum<vi>, "Value"=w612:T2)  [unwired: 1 in, 1 out]
            n225 = property class="DigNum (strict)"(reference=w617, "Value"=w616) -> (reference out=w615:refnum<vi>)  [unwired: 1 in, 1 out]
            n226 = Bundle By Name(cluster=w612, "Vehicle Out of Position"=FALSE, "Air Dry"=TRUE ("Under Body Wash")) -> (w611:T2)
            n227 = case shown="False" w623 {
              tunnel: w622 -> [w624 w631]
              tunnel: [w624 w630] -> w621
              tunnel: ["Air Dry" ""] -> w620
              tunnel: w615 -> [_ w627]
              frame False {
              }
              frame True {
                n228 = call "Timer.vi"("entrée d'erreur"=w631, "State"=Time."Start") -> ("sortie d'erreur"=w630:errorcluster, "Elapsed"=w629:dbl)  [unwired: 7 in, 1 out]
                n229 = property class="DigNum (strict)"(reference=w627, "Value"=w629) -> ()  [unwired: 1 in, 2 out]
              }
            }
            n230 = property class="Clust (strict)"(reference=w610, "Value"=w611) -> ()  [unwired: 1 in, 2 out]
          }
          frame 0..2 {
            n231 = property class="Clust (strict)"(reference=w632) -> (reference out=w633:refnum<vi>, "Value"=w635:T2)  [unwired: 1 in, 1 out]
            n232 = call "Timer.vi"("entrée d'erreur"=w639, "State"=Time."Pause") -> ("sortie d'erreur"=w638:errorcluster, "Elapsed"=w641:dbl)  [unwired: 7 in, 1 out]
            n233 = Bundle By Name(cluster=w635, "Vehicle Out of Position"=TRUE) -> (w634:T2)
            n234 = property class="DigNum (strict)"(reference=w642, "Value"=w641) -> ()  [unwired: 1 in, 2 out]
            n235 = property class="Clust (strict)"(reference=w633, "Value"=w634) -> ()  [unwired: 1 in, 2 out]
          }
        }
        n236 = call <vilib>:"Add State(s) to Queue__JKI_lib_State_Machine.vi"("State(s) in Front (\"\")"=w602, "State(s) in (\"\")"=w608) -> ("States Out"=w607:string)  [unwired: 13 in]
      }
      frame "Exi" {
        # "Your code here.\n(You can make a copy of, or modify, this frame)"
        n237 = Unbundle By Name(w650) -> ("Car Wash Indicators"=w645:refnum<vi>, "Wash Entry"=w644:refnum<vi>, "Elapsed Time"=w646:refnum<vi>)
        n238 = case shown="4, Default" w649 {
          tunnel: [w665 w672] -> w647
          tunnel: w646 -> [w662 w676]
          tunnel: ["" "Exi"] -> w643
          tunnel: w648 -> [w663 w673]
          tunnel: w645 -> [w661 w666]
          tunnel: w644 -> [w660 _]
          frame 4, Default {
            w655 = FALSE ("Car Wash Indicators.Under Body Wash")
            n239 = property class="Bool (strict)"(reference=w660, "Value"=FALSE) -> ()  [unwired: 1 in, 2 out]
            n240 = property class="Clust (strict)"(reference=w661) -> (reference out=w653:refnum<vi>, "Value"=w656:T2)  [unwired: 1 in, 1 out]
            n241 = Bundle By Name(cluster=w656, "Under Body Wash"=w655, "Bug Remover"=w655, "Pre-Soak"=w655, "High Pressure Wash"=w655, "Low Pressure Wax"=w655, "Spot Free Rinse"=w655, "Tire Shine Foam"=w655, "Air Dry"=w655, "Vehicle Out of Position"=w655) -> (w657:T2)
            n242 = call "Timer.vi"("entrée d'erreur"=w663, "State"=Time."Start") -> ("sortie d'erreur"=w665:errorcluster, "Elapsed"=w659:dbl)  [unwired: 7 in, 1 out]
            n243 = property class="DigNum (strict)"(reference=w662, "Value"=w659) -> ()  [unwired: 1 in, 2 out]
            n244 = property class="Clust (strict)"(reference=w653, "Value"=w657) -> ()  [unwired: 1 in, 2 out]
          }
          frame 0..3 {
            n245 = property class="Clust (strict)"(reference=w666) -> (reference out=w667:refnum<vi>, "Value"=w669:T2)  [unwired: 1 in, 1 out]
            n246 = call "Timer.vi"("entrée d'erreur"=w673, "State"=Time."Pause") -> ("sortie d'erreur"=w672:errorcluster, "Elapsed"=w675:dbl)  [unwired: 7 in, 1 out]
            n247 = Bundle By Name(cluster=w669, "Vehicle Out of Position"=TRUE) -> (w668:T2)
            n248 = property class="DigNum (strict)"(reference=w676, "Value"=w675) -> ()  [unwired: 1 in, 2 out]
            n249 = property class="Clust (strict)"(reference=w667, "Value"=w668) -> ()  [unwired: 1 in, 2 out]
          }
        }
        n250 = call <vilib>:"Add State(s) to Queue__JKI_lib_State_Machine.vi"("State(s) in Front (\"\")"=w643, "State(s) in (\"\")"=w652) -> ("States Out"=w651:string)  [unwired: 13 in]
      }
    }
  }
